vi "LEBITplc.SetPLC.vi"(0 "i ref in":refnum<vi>, 1 "CommandName":string, 2 "Binary Selection":i16, 3 "Value":dbl, 4 "log?":bool, 5 "error IO":errorcluster, 7 "index of element":i32) -> (14 "i ref out":refnum<vi>, 19 "error out":errorcluster)   [LabVIEW 2014, in "LEBITplc.lvlib"]
uses:
  LEBITplc.lvlib
  CS_Core/CSSystem/CoreDefs/CoreDefs.error_type.ctl
  CS_Core/CSSystem/CoreDefs/CoreDefs.error_severity.ctl
  CS_Core/CSSystem/CoreLib/CoreLib.lvlib
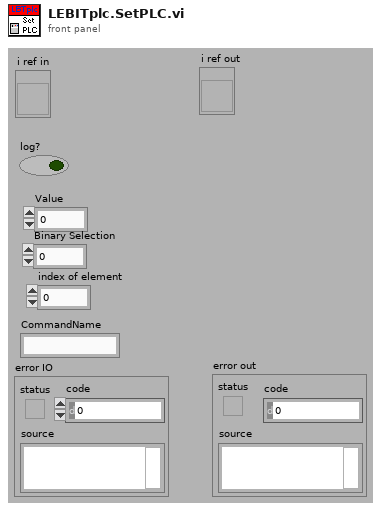
[diagram p1: front panel]
types:
  T1 = typedef "CoreDefs.error_severity.ctl" = enum16{"undefined", "information", "warning", "error", "fatal"}
  T2 = typedef "CoreDefs.error_type.ctl" = enum16{"no error", "can't load process", "can't unload process", "process does not exist", "can't install process", "can't remove process", "unknown function", "time out", "can't execute function", "duplicate queue name", "super not found", "caller queue invalid", "can't ping process", "unknown error", "VISA Error", "VISA timeout", "GPIB timeout", "GPIB error", "communication error", "data type mismatch", "can't read data from OPC server", "can't write data to OPC server", "OET error", "function not implemented", "process already exists", "invalid Shared Variable name", "error writing Shared Variable", "error reading Shared Variable", "invalid client name", "corrupt database", "unknown class", "call not authorized", "parameter out of range", "OET timeout: can't get data to modify", "invalid queue name", "requested operation incompatible with current state", "event undefined", "event disabled", "state undefined", "caller is not a friend", "EventBuilder: bad eventID", "EventBuilder: no DAQ devices", "a thread must not stop itself", "UNUSED ELEMENT4", "DiscArchiver: eventData incomplete", "DiscArchiver: eventData does not belong to run", "DiscArchiver: can't open file", "DiscArchiver: can't write to file", "DiscArchiver: available disc space low", "can't acquire semaphore", "error reading data from database", "notifier object is not existing", "can't register process", "can't unregister process", "illegal event type", "object disabled", "object already exists", "can't change state", "Instrument not found", "no connection to remote node", "invalid reference", "N/A", "UNUSED ELEMENT 1", "element not found", "illegal TCP/IP connection detected", "object does not exist", "invalid access ID", "unknown CS system", "invalid privilige", "unsupported data type", "unsupported server type", "IO server already exists", "Shared Variable already exists"}
  T3 = typedef "LEBITplc.lvlib/LEBITplc.i attribute.ctl" = cluster{"LLFLocation":string, "SetFileLocation":string, "nickNames":string[], "setValuePLCServiceID":i32[], "GUIServiceID":i32[], "monValuePLC":string[], "SetValueServiceID":i32[], "MonValueServiceID":i32[], "SetValue":dbl[][], "SetValueMin":dbl[], "SetValueMax":dbl[], "SetValueInfoServiceID":i32[], "GUINames":string[], "ListOfBases":string[], "Scale":dbl[], "Offset":dbl[], "setValuePLC":string[], "BaseName":string[], "ScaleServiceID":i32[], "OffsetServiceID":i32[], "AllPLCValues":string[], "CondSpecialArray":string[][], "CondSpecialIndex":i32[], "CondSpecialMonValue":dbl[], "RecentlyChanged":i32[], "SetFileLocationID":i32, "Dependent-Monitors":string[][], "LastLoadedFiles":string[], "IonGuideCalibLocation":string, "Monitor Dependent":string[], "Special":string[], "PLC?":bool[], "Start Date":string, "ListOfBasesServiceID":i32, "SETRA VISA resource":refnum<visa-resource-name>}
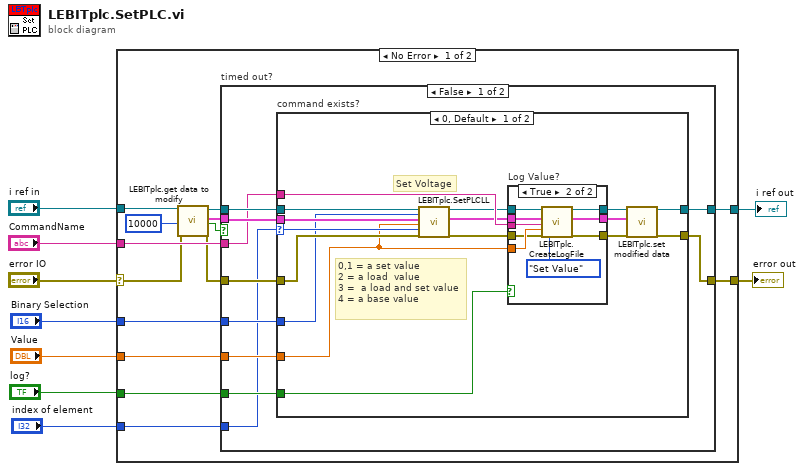
[diagram p0: block diagram]
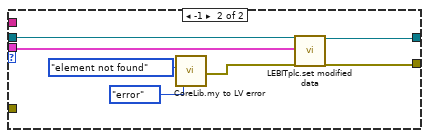
[diagram p3: hidden frame]
diagram:
  n1 = case shown="No Error" "error IO" {
    selector: "error IO" -> [w17 w71]
    tunnel: "CommandName" -> [w22 _]
    tunnel: "i ref in" -> [w20 w72]
    tunnel: [w19 w71] -> w7
    tunnel: [w18 w72] -> w6
    tunnel: "log?" -> [w13 _]
    tunnel: "Value" -> [w12 _]
    tunnel: "Binary Selection" -> [w11 _]
    tunnel: "index of element" -> [w10 _]
    frame No Error {
      n2 = call "LEBITplc.get data to modify.vi"("i ref in"=w20, "ms timeout (10000)"=10000, "error in (no error)"=w17) -> ("i ref out"=w21:refnum<vi>, "i attribute"=w23:T3, "timed out"=w15:bool, "error out"=w14:errorcluster)  [unwired: 13 in]
      n3 = case "timed out?" shown="False" w15 {
        tunnel: w23 -> [w33 _]
        tunnel: w22 -> [w28 _]
        tunnel: w21 -> [w32 w70]
        tunnel: [w30 w69] -> w19
        tunnel: [w29 w70] -> w18
        tunnel: w14 -> [w31 w69]
        tunnel: w13 -> [w27 _]
        tunnel: w12 -> [w26 _]
        tunnel: w11 -> [w25 _]
        tunnel: w10 -> [w24 _]
        frame False {
          n4 = case "command exists?" shown="0, Default" w24 {
            selector: w24 -> [w44 _]
            tunnel: [w48 w65] -> w29
            tunnel: [w49 w62] -> w30
            tunnel: w32 -> [w47 w66]
            tunnel: w33 -> [w46 w64]
            tunnel: w31 -> [w45 _]
            tunnel: w28 -> [w43 _]
            tunnel: w27 -> [w42 _]
            tunnel: w26 -> [w41 _]
            tunnel: w25 -> [w34 _]
            frame 0, Default {
              # "Set Voltage"
              # "0,1 = a set value\n2 = a load  value\n3 =  a load and set value\n4 = a base value"
              n5 = call "LEBITplc.SetPLCLL.vi"("i ref in"=w47, "Binary Selection"=w34, "i attribute in"=w46, "Value"=w41, "index of element"=w44, "error IO"=w45) -> ("i ref out"=w39:refnum<vi>, "i attribute out"=w38:T3, "error out"=w40:errorcluster)  [unwired: 11 in]
              n6 = case "Log Value?" shown="True" w42 {
                tunnel: w43 -> [_ w61]
                tunnel: w41 -> [_ w60]
                tunnel: w40 -> [w52 w59]
                tunnel: [w52 w58] -> w36
                tunnel: w39 -> [w51 w56]
                tunnel: [w51 w57] -> w37
                tunnel: w38 -> [w50 w54]
                tunnel: [w50 w55] -> w35
                frame False {
                }
                frame True {
                  n7 = call "LEBITplc.CreateLogFile.vi"("i ref in"=w56, "i attribute in"=w54, "nickName"=w61, "value\nnobase"=w60, "error in"=w59, "Enum"=enum16{"Set Value", "Loaded File"}."Set Value") -> ("i ref out"=w57:refnum<vi>, "i attribute out"=w55:T3, "error out"=w58:errorcluster)  [unwired: 11 in]
                }
              }
              n8 = call "LEBITplc.set modified data.vi"("i ref in"=w37, "i attribute"=w35, "error in (no error)"=w36) -> ("i ref out"=w48:refnum<vi>, "error out"=w49:errorcluster)  [unwired: 15 in]
            }
            frame -1 {
              n9 = call "CoreLib.my to LV error.vi"("ErrorTypes"=CoreDefs.error_type."element not found", "severityLevel"=CoreDefs.error_severity."error") -> ("myErrorCluster"=w63:errorcluster)  [unwired: 16 in, 1 out]
              n10 = call "LEBITplc.set modified data.vi"("i ref in"=w66, "i attribute"=w64, "error in (no error)"=w63) -> ("i ref out"=w65:refnum<vi>, "error out"=w62:errorcluster)  [unwired: 15 in]
            }
          }
        }
        frame True {
        }
      }
    }
    frame Error {
    }
  }
  "error out" <- w7
  "i ref out" <- w6
